vi "Get All VIs in Memory Including statically-referenced Reentrant Clones.vi"(8 "error in (no error)":errorcluster, 11 "App Refnum":refnum<vi>) -> (0 "error out":errorcluster, 1 "Number Of VIs in Memory":i32, 2 "All VIs in Memory Including Reentrant Clones":string[](array[string]), 3 "App Refnum Out":refnum<vi>, 4 "run time (sec)":dbl)   [LabVIEW 2013, in "LVTM.lvlib"]
doc: "This VI will return a list of all VIs currently in memory, including all statically-referenced reentrant clones. The names of any Custom Probes currently in memory will be excluded."
uses:
  LVTM.lvlib
panel:
  in  "Ignore DepCache":bool
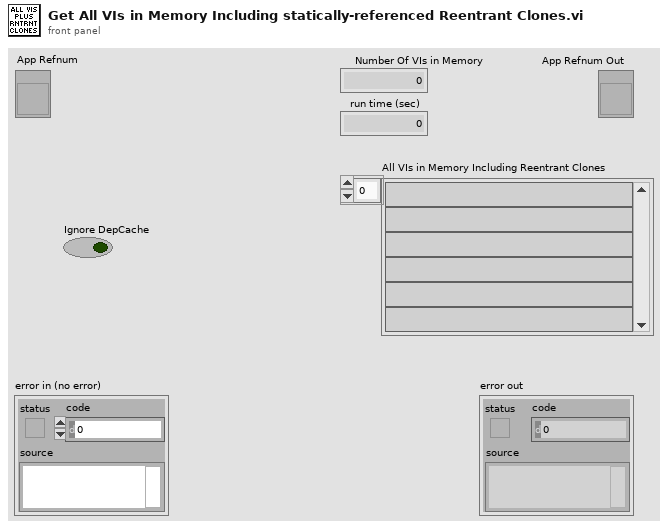
[diagram p1: front panel]
types:
  T1 = enum8{"Include the clone VI", "Include the original reentrant VI instead of the clone VI", "Include both the original reentrant VI and the clone VI"}
  T2 = enum32{"invalid VI type", "Standard VI", "Control VI", "Global VI", "Polymorphic VI", "Configuration VI", "SubSystem", "Facade VI", "Method VI", "Statechart Diagram VI"}
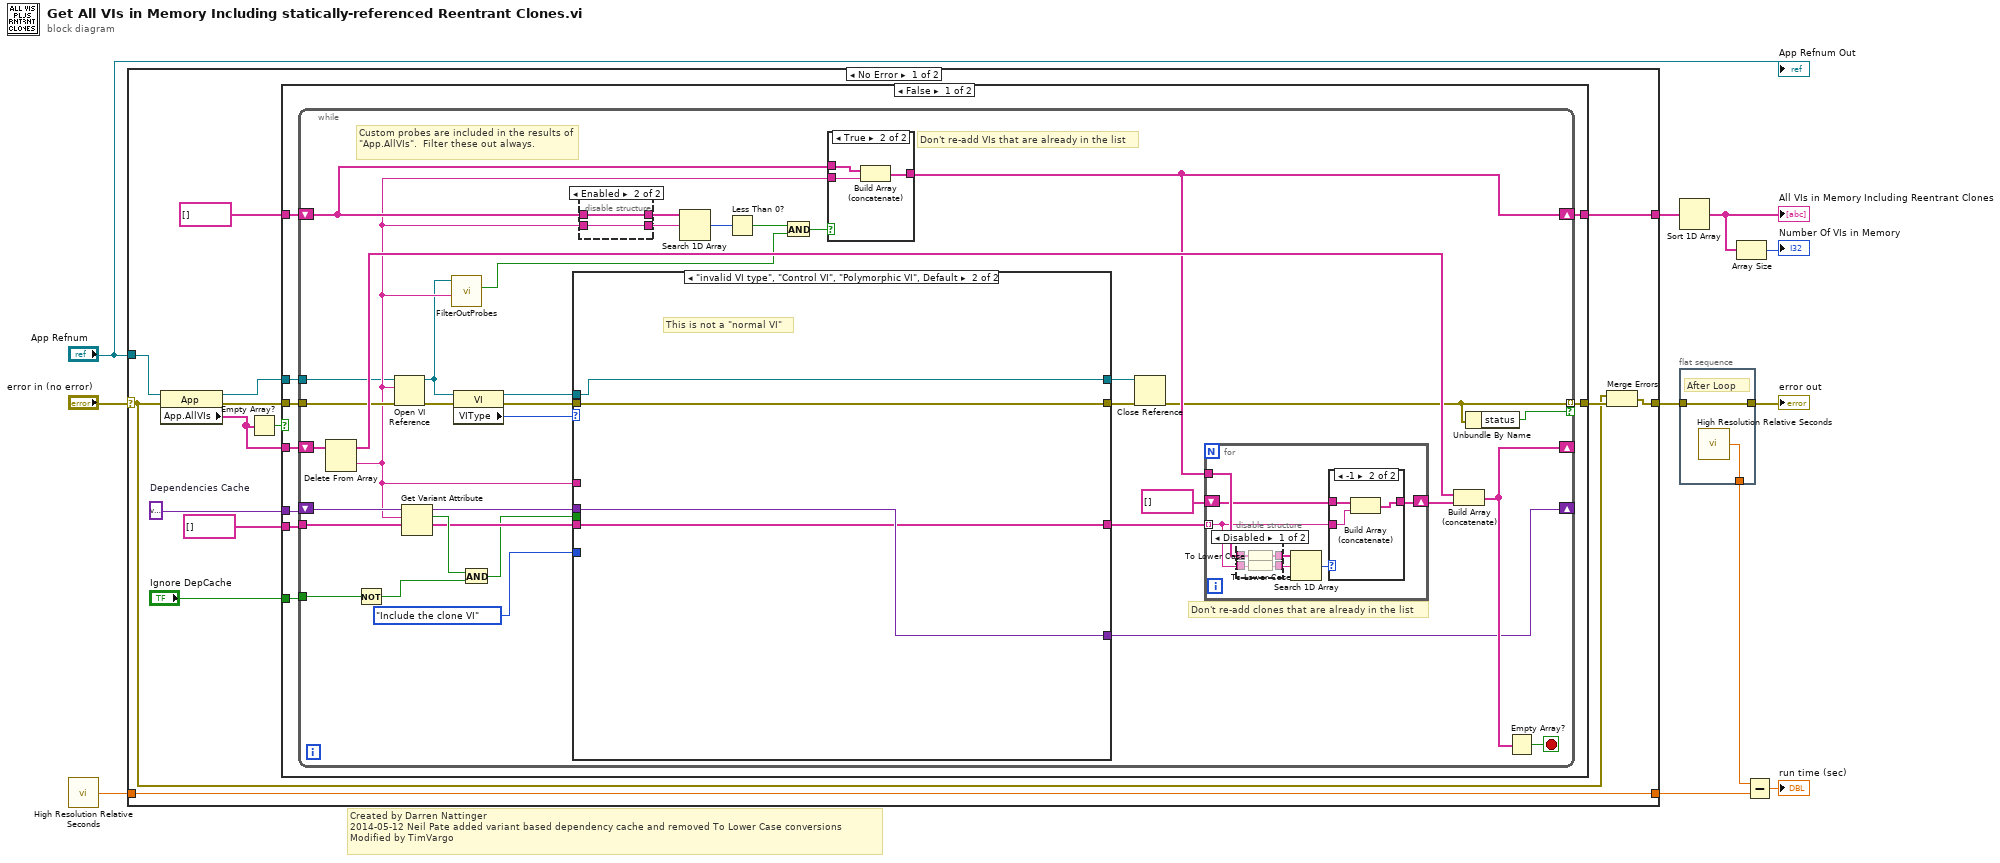
[diagram p0: block diagram]
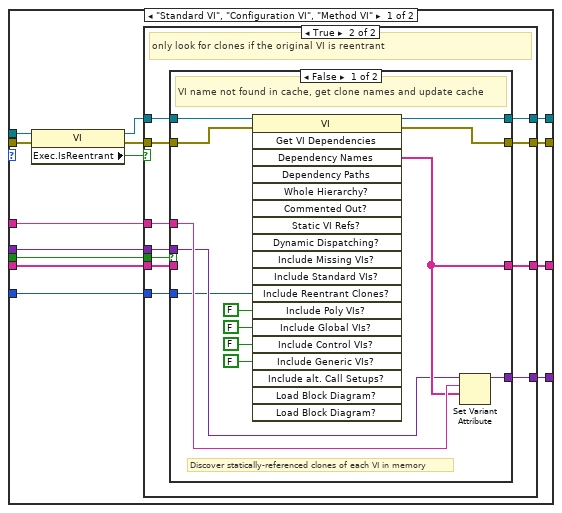
[diagram p2: hidden frame]
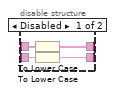
[diagram p5: hidden frame]
diagram:
  # "Created by Darren Nattinger\n2014-05-12 Neil Pate added variant based dependency cache and removed To Lower Case conversions\nModified by TimVargo"
  n1 = call <vilib>:"High Resolution Relative Seconds.vi"() -> ("relative seconds"=w4:dbl)
  n2 = case shown="No Error" "error in (no error)" {
    selector: "error in (no error)" -> [w15 w151]
    tunnel: [w16 w151] -> w6
    tunnel: "App Refnum" -> [w14 _]
    tunnel: [w22 _] -> w10
    tunnel: w4 -> [w20 w150]
    tunnel: [w20 w150] -> w3
    frame No Error {
      w18 = variant  # Dependencies Cache
      n3 = property class="App"(reference=w14, error in=w15) -> (reference out=w24:refnum<vi>, error out=w25:errorcluster, "App.AllVIs"=w12:string[])
      n4 = Empty Array?(array=w12) -> (empty?=w13:bool)
      n5 = case shown="False" w13 {
        tunnel: w25 -> [w34 _]
        tunnel: w24 -> [w33 _]
        tunnel: w12 -> [w32 _]
        tunnel: string[] [] -> [w31 w149]
        tunnel: [w30 w149] -> w22
        tunnel: [w29 _] -> w21
        tunnel: string[] [] -> [w28 _]
        tunnel: w18 -> [w27 _]
        tunnel: "Ignore DepCache" -> [w26 _]
        frame False {
          n6 = while {
            tunnel: w33 -> [w51]
            shift-right: [w69] -> _
            shift-left: w32 -> [w71]
            shift-right: [w63] -> w30
            shift-left: w31 -> [w64]
            tunnel: w28 -> [w62]
            shift-right: [w59] -> _
            shift-left: w27 -> [w61]
            tunnel: w26 -> [w48]
            tunnel: w34 -> [w53]
            tunnel: [w46] -> w29 mode=indexing if=w45
            stop <- w49 stop-if-true
            # "Don't re-add VIs that are already in the list"
            # "Custom probes are included in the results of \"App.AllVIs\".  Filter these out always."
            # "Don't re-add clones that are already in the list"
            n7 = Delete From Array(array=w71) -> (deleted portion=w52:string, array with subset deleted=w70:string[])  [unwired: 2 in]
            n8 = Not(x=w48) -> (.not. x?=w47:bool)
            n9 = Open VI Reference(application reference (local)=w51, vi path=w52, error in (no error)=w53) -> (vi reference=w44:refnum<vi>, error out=w42:errorcluster)  [unwired: 3 in]
            n10 = Get Variant Attribute(Variant=w61, name=w52, default value (empty Variant)=w62) -> (duplicate Variant=w38:variant, found=w40:bool, value=w39:string[])  [unwired: 1 in, 1 out]
            n11 = call "FilterOutProbes.vi"("VI reference in"=w44, "Item Name"=w52) -> ("NotAProbe"=w55:bool)  [unwired: 7 in, 1 out]
            n12 = property class="VI"(reference=w44, error in=w42) -> (reference out=w43:refnum<vi>, error out=w41:errorcluster, "VIType"=w35:T2)
            n13 = And(x=w40, y=w47) -> (x .and. y?=w36:bool)
            n14 = case shown="\"invalid VI type\", \"Control VI\", \"Polymorphic VI\", Default" w35 {
              tunnel: [w85 w119] -> w60
              tunnel: [w84 w121] -> w59
              tunnel: [w83 w118] -> w54
              tunnel: w52 -> [w82 _]
              tunnel: [w81 w120] -> w50
              tunnel: w43 -> [w80 w118]
              tunnel: w41 -> [w79 w120]
              tunnel: w39 -> [w78 w119]
              tunnel: w38 -> [w77 w121]
              tunnel: T1."Include the clone VI" ("Include Reentrant Clones?") -> [w76 _]
              tunnel: w36 -> [w72 _]
              frame "Standard VI", "Configuration VI", "Method VI" {
                n15 = property class="VI"(reference=w80, error in=w79) -> (reference out=w73:refnum<vi>, error out=w75:errorcluster, "Exec.IsReentrant"=w74:bool)
                n16 = case shown="True" w74 {
                  tunnel: [w87 w100] -> w85
                  tunnel: w72 -> [_ w99]
                  tunnel: w78 -> [w87 w98]
                  tunnel: w77 -> [w86 w97]
                  tunnel: [w86 w96] -> w84
                  tunnel: w76 -> [_ w95]
                  tunnel: [w89 w94] -> w83
                  tunnel: w75 -> [w88 w93]
                  tunnel: w82 -> [_ w92]
                  tunnel: w73 -> [w89 w91]
                  tunnel: [w88 w90] -> w81
                  frame False {
                    # "the original VI is not reentrant"
                  }
                  frame True {
                    # "only look for clones if the original VI is reentrant"
                    n17 = case shown="False" w99 {
                      tunnel: w93 -> [w101 w117]
                      tunnel: [w103 w117] -> w90
                      tunnel: w92 -> [w109 _]
                      tunnel: [w108 w116] -> w100
                      tunnel: w98 -> [_ w116]
                      tunnel: w97 -> [w107 w115]
                      tunnel: [w106 w115] -> w96
                      tunnel: w95 -> [w105 _]
                      tunnel: w91 -> [w102 w114]
                      tunnel: [w104 w114] -> w94
                      frame False {
                        # "Discover statically-referenced clones of each VI in memory"
                        # "VI name not found in cache, get clone names and update cache"
                        n18 = invoke class="VI" method="Get VI Dependencies"(reference=w102, error in=w101, "Include Reentrant Clones?"=w105, "Include Poly VIs?"=FALSE, "Include Global VIs?"=FALSE, "Include Control VIs?"=FALSE, "Include Generic VIs?"=FALSE) -> (reference out=w104:refnum<vi>, error out=w103:errorcluster, "Dependency Names"=w108:string[])  [unwired: 12 in, 16 out]
                        n19 = Set Variant Attribute(Variant=w107, name=w109, value=w108) -> (Variant out=w106:variant)  [unwired: 1 in, 2 out]
                      }
                      frame True {
                        # "VI name found in cache, use dependencies from cache"
                      }
                    }
                  }
                }
              }
              frame "invalid VI type", "Control VI", "Polymorphic VI", Default {
                # "This is not a \"normal VI\""
              }
            }
            n20 = disable-structure shown="Enabled" {
              disable-tunnel: [w125 w126] -> w66
              disable-tunnel: [w124 w127] -> w65
              disable-tunnel: w64 -> [w123 w127]
              disable-tunnel: w52 -> [w122 w126]
              frame Disabled {
                n21 = To Lower Case(string=w123) -> (all lower case string=w124:string[])
                n22 = To Lower Case(string=w122) -> (all lower case string=w125:string)
              }
              frame Enabled {
              }
            }
            n23 = Search 1D Array(1D array=w65, element=w66) -> (index of element=w56:i32)  [unwired: 1 in]
            n24 = Less Than 0?(x=w56) -> (x < 0?=w57:bool)
            n25 = And(x=w57, y=w55) -> (x .and. y?=w58:bool)
            n26 = case shown="True" w58 {
              tunnel: w64 -> [w128 w131]
              tunnel: w52 -> [_ w130]
              tunnel: [w128 w129] -> w63
              frame False {
              }
              frame True {
                n27 = Build Array (concatenate)(w131, w130) -> (w129:string[])
              }
            }
            n28 = Close Reference(reference=w54, error in (no error)=w50) -> (error out=w46:errorcluster)
            n29 = for {
              tunnel: w63 -> [w138]
              tunnel: w60 -> [w133] mode=indexing
              shift-right: [w134] -> w67
              shift-left: string[] [] -> [w135]
              n30 = disable-structure shown="Disabled" {
                disable-tunnel: w138 -> [w142 w144]
                disable-tunnel: [w141 w143] -> w137
                disable-tunnel: w133 -> [w140 w143]
                disable-tunnel: [w139 w144] -> w132
                frame Disabled {
                  n31 = To Lower Case(string=w142) -> (all lower case string=w139:string[])
                  n32 = To Lower Case(string=w140) -> (all lower case string=w141:string)
                }
                frame Enabled {
                }
              }
              n33 = Search 1D Array(1D array=w132, element=w137) -> (index of element=w136:i32)  [unwired: 1 in]
              n34 = case shown="-1" w136 {
                tunnel: w135 -> [w145 w148]
                tunnel: [w145 w147] -> w134
                tunnel: w133 -> [_ w146]
                frame Default {
                }
                frame -1 {
                  n35 = Build Array (concatenate)(w148, w146) -> (w147:string[])
                }
              }
            }
            n36 = Build Array (concatenate)(w70, w67) -> (w69:string[])
            n37 = Unbundle By Name(w46) -> ("status"=w45:bool)
            n38 = Empty Array?(array=w69) -> (empty?=w49:bool)
          }
        }
        frame True {
        }
      }
      n39 = Merge Errors(w15, w21) -> (w16:errorcluster)
    }
    frame Error {
    }
  }
  n40 = Sort 1D Array(array=w10) -> (sorted array=w8:string[])
  "All VIs in Memory Including Reentrant Clones" <- w8
  n41 = flat-sequence {
    tunnel: w6 -> [w153]
    tunnel: [w153] -> w5
    tunnel: [w152] -> w1
    frame #0 {
      # "After Loop"
      n42 = call <vilib>:"High Resolution Relative Seconds.vi"() -> ("relative seconds"=w152:dbl)
    }
  }
  n43 = Array Size(array=w8) -> (size(s)=→"Number Of VIs in Memory":i32)
  n44 = Subtract(x=w1, y=w3) -> (x-y=→"run time (sec)":dbl)
  "error out" <- w5
  "App Refnum Out" <- "App Refnum"
